vi "AlphaValve_control.vi"(4 "FieldPoint IO Point":refnum<k21>, 6 "reference in":refnum<vi>, 7 "OK Button 8":bool, 9 "FieldPoint IO Point 2":refnum<k21>, 10 "FieldPoint IO Point 3":refnum<k21>, 11 "Boolean in":refnum<vi>) -> (0 "error out":errorcluster, 1 "Alpha Open":errorcluster caption="error out", 2 "Alpha Close":errorcluster caption="error out", 3 "Boolean 10":bool, 5 "Boolean 13":bool)   [LabVIEW 2014]
uses:
  <vilib>/FieldPoint/Polymorphic Write.llb/FP Write (Boolean -IO).vi
  <vilib>/FieldPoint/Polymorphic Read.llb/FP Read (Boolean -IO).vi
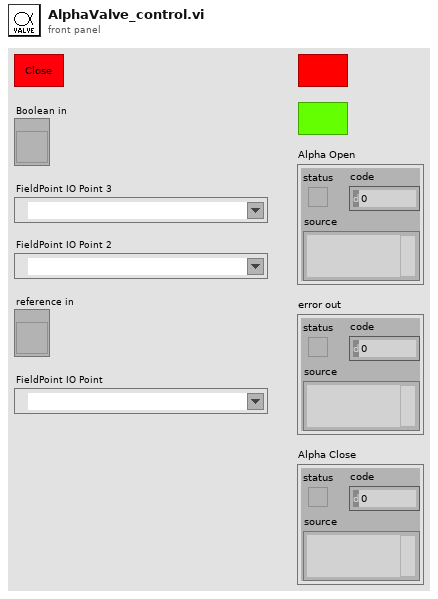
[diagram p1: front panel]
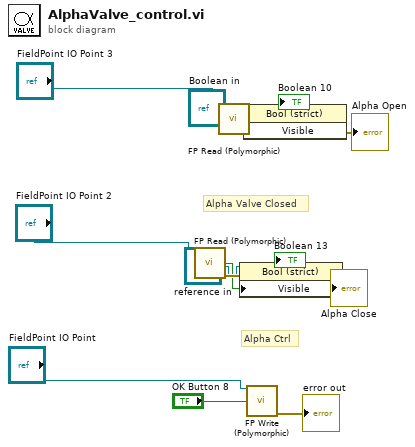
[diagram p0: block diagram]
diagram:
  # "Alpha Ctrl"
  # "Alpha Valve Closed"
  n1 = call-poly <vilib>:"FP Read (Polymorphic).vi"("FieldPoint IO Point In"="FieldPoint IO Point 2") -> ("value"=w8:bool, "error out"=w11:errorcluster)  [unwired: 11 in, 2 out]
  n2 = call-poly <vilib>:"FP Read (Polymorphic).vi"("FieldPoint IO Point In"="FieldPoint IO Point 3") -> ("value"=w7:bool, "error out"=w9:errorcluster)  [unwired: 11 in, 2 out]
  n3 = property on="Property Node" class="Bool (strict)"(reference="reference in", error in=w11, "Visible"=w8) -> (error out=→"Alpha Close":errorcluster)  [unwired: 1 out]
  n4 = property on="Property Node" class="Bool (strict)"(reference="Boolean in", error in=w9, "Visible"=w7) -> (error out=→"Alpha Open":errorcluster)  [unwired: 1 out]
  n5 = call-poly <vilib>:"FP Write (Polymorphic).vi"("FieldPoint IO Point In"="FieldPoint IO Point", "value"="OK Button 8") -> ("error out"=→"error out":errorcluster)  [unwired: 11 in, 2 out]
